vi "Rx Async.vi"(8 "error in (no error)":errorcluster, 10 "Dispatcher Interface in":refnum<class "Dispatcher Interface.lvclass">, 11 "Plugin in":refnum<class "Plugin.lvclass">) -> (0 "error out":errorcluster, 2 "Dispatcher Interface out":refnum<class "Dispatcher Interface.lvclass">, 3 "Plugin out":refnum<class "Plugin.lvclass">)   [LabVIEW 2017, in "DSF Core.lvlib" / "Plugin.lvclass"]
uses:
  Plugin.lvclass
  Interfaces/Dispatcher/Dispatcher Interface.lvclass
  C:/Git/DSF/Data Sharing Framework Core/Classes/Interfaces/Interface/Interface.lvclass
  Plugin.lvclass/Plugin.ctl
  Transfer Group/Transfer Group.lvclass/Transfer Group.ctl
  Timing/Timing.lvclass/Timing.ctl
  Interfaces/Dispatcher/Command.ctl
  Buffers/Buffers.lvclass/Buffers.ctl
  Interfaces/Interface/Interface.lvclass/Interface.ctl
  Interfaces/Dispatcher/Send Dispatcher Command.vi
  Transfer Group/Retrieve from FIFO.vi
  Transfer Group Status/Write Status.vi
  Interfaces/Dispatcher/Write.vi
  Interfaces/Dispatcher/Write Dispatcher Command.vi
  Transfer Group/Read Return FIFO.vi
  Transfer Group/Increment Late Count.vi
  Transfer Group Status/Status Size.vi
  Interfaces/Interface/Send Command.vi
  Interfaces/Interface/Write RT FIFO.vi
  Buffer/Buffer.lvclass
  C:/Git/DSF/LabVIEW-Memory/Source/Classes/Pointer/Pointer.lvclass
  Transfer Group Status/Status.lvclass
  LabVIEW-Memory/Source/Classes/Pointer/Get Address.vi
  LabVIEW-Memory/Source/Classes/Pointer/Check Size.vi
  LabVIEW-Memory/Source/Classes/Pointer/Check Null Pointer.vi
  Interfaces/Interface/Errors.vi
  Interfaces/Dispatcher/Command Timeout.vi
  VIs/VI Name.vi
  Interfaces/Dispatcher/Class Name.vi
  LabVIEW-Memory/Source/Classes/Pointer/Copy All.vi
  Transfer Group/Errors.vi
  Transfer Group/Return Timeout Error.vi
  Transfer Group/Invalid Iteration Error.vi
  Transfer Group/Transfer Group.lvclass
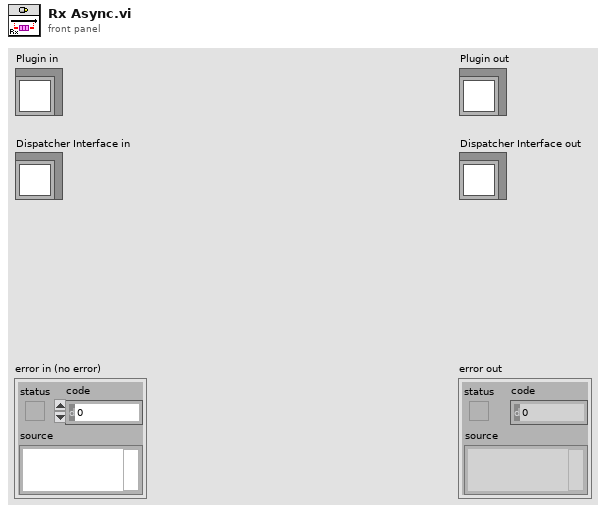
[diagram p1: front panel]
types:
  T1 = typedef "DSF Core.lvlib/Dispatcher Interface.lvclass/Command.ctl" = enum8{"Rx", "Tx", "Set Inline Buffer", "Shutdown"}
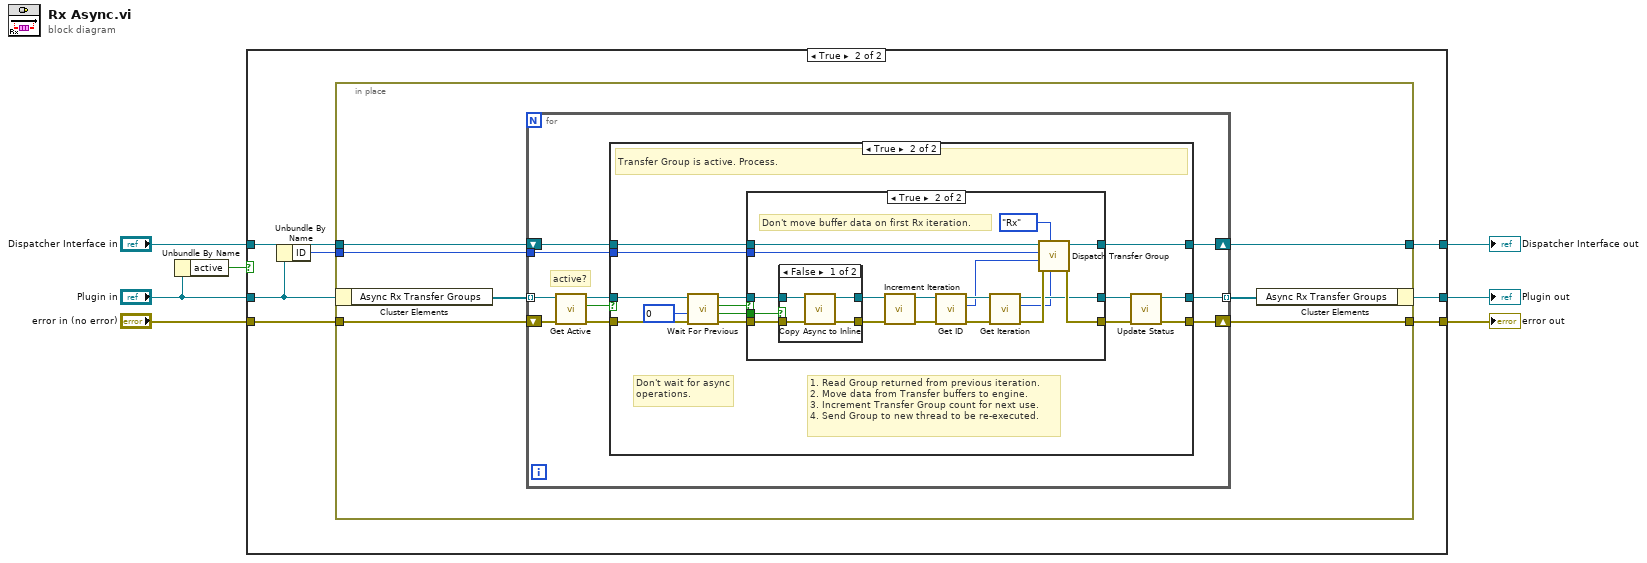
[diagram p0: block diagram]
diagram:
  n1 = Unbundle By Name("Plugin in") -> ("active"=w1:bool)
  n2 = case shown="True" w1 {
    tunnel: "error in (no error)" -> [w8 w17]
    tunnel: [w8 w16] -> w6
    tunnel: [w10 w15] -> w5
    tunnel: "Dispatcher Interface in" -> [w9 w14]
    tunnel: [w9 w13] -> w3
    tunnel: "Plugin in" -> [w10 w12]
    frame False {
    }
    frame True {
      n3 = Unbundle By Name(w12) -> ("ID"=w11:i32)
      n4 = in-place {
        in-place-border: w17 -> [w24]
        in-place-border: [w23] -> w16
        in-place-border: w14 -> [w20]
        in-place-border: [w19] -> w13
        in-place-border: w11 -> [w18]
        n5 = in-place-cluster #1(w12) -> ("Async Rx Transfer Groups"=w22:refnum<class "Transfer Group.lvclass">[])
        n6 = for {
          tunnel: w22 -> [w27] mode=indexing
          shift-right: [w33] -> w23
          shift-left: w24 -> [w32]
          tunnel: [w31] -> w21 mode=indexing
          shift-right: [w29] -> w19
          shift-left: w20 -> [w30]
          tunnel: w18 -> [w28]
          # "active?"
          n7 = call "Get Active.vi"("Transfer Group in"=w27) -> ("active"=w25:bool, "Transfer Group out"=w26:refnum<class "Transfer Group.lvclass">)  [unwired: 9 in]
          n8 = case shown="True" w25 {
            tunnel: [w36 w39] -> w33
            tunnel: w32 -> [w36 w49]
            tunnel: w26 -> [w35 w50]
            tunnel: [w35 w38] -> w31
            tunnel: w30 -> [w34 w44]
            tunnel: [w34 w45] -> w29
            tunnel: w28 -> [_ w43]
            frame False {
              # "Transfer Group is not active. Skip."
            }
            frame True {
              # "Don't wait for async operations."
              # "1. Read Group returned from previous iteration.\n2. Move data from Transfer buffers to engine.\n3. Increment Transfer Group count for next use.\n4. Send Group to new thread to be re-executed."
              # "Transfer Group is active. Process."
              n9 = call "Wait For Previous.vi"("error in (no error)"=w49, "timeout in ms (0)"=0, "Transfer Group in"=w50) -> ("error out"=w46:errorcluster, "first iteration"=w37:bool, "ready for next"=w42:bool, "Transfer Group out"=w47:refnum<class "Transfer Group.lvclass">)  [unwired: 5 in]
              n10 = case shown="True" w42 {
                tunnel: w47 -> [w53 w70]
                tunnel: [w53 w59] -> w41
                tunnel: [w52 w60] -> w40
                tunnel: w46 -> [w52 w69]
                tunnel: [w51 w57] -> w45
                tunnel: w44 -> [w51 w56]
                tunnel: w43 -> [_ w55]
                tunnel: w37 -> [_ w54]
                frame False {
                }
                frame True {
                  # "Don't move buffer data on first Rx iteration."
                  n11 = case shown="False" w54 {
                    tunnel: w70 -> [w74 w76]
                    tunnel: w69 -> [w73 w75]
                    tunnel: [w72 w76] -> w62
                    tunnel: [w71 w75] -> w61
                    frame False {
                      n12 = call "Copy Async to Inline.vi"("error in (no error)"=w73, "Transfer Group in"=w74) -> ("error out"=w71:errorcluster, "Transfer Group out"=w72:refnum<class "Transfer Group.lvclass">)  [unwired: 8 in]
                    }
                    frame True {
                    }
                  }
                  n13 = call "Increment Iteration.vi"("error in (no error)"=w61, "Transfer Group in"=w62) -> ("error out"=w66:errorcluster, "Transfer Group out"=w68:refnum<class "Transfer Group.lvclass">)  [unwired: 8 in]
                  n14 = call "Get ID.vi"("Transfer Group in"=w68) -> ("id"=w65:i32, "Transfer Group out"=w67:refnum<class "Transfer Group.lvclass">)  [unwired: 9 in]
                  n15 = call "Get Iteration.vi"("error in (no error)"=w66, "Transfer Group in"=w67) -> ("error out"=w64:errorcluster, "iteration"=w58:u64, "Transfer Group out"=w59:refnum<class "Transfer Group.lvclass">)  [unwired: 7 in]
                  n16 = call "Dispatch Transfer Group.vi"("Iteration"=w58, "command"=Command."Rx", "error in (no error)"=w64, "Transfer Group ID"=w65, "Plugin ID"=w55, "Dispatcher Interface in"=w56) -> ("error out"=w60:errorcluster, "Dispatcher Interface out"=w57:refnum<class "Dispatcher Interface.lvclass">)  [unwired: 4 in]
                }
              }
              n17 = call "Update Status.vi"("error in (no error)"=w40, "Transfer Group in"=w41) -> ("error out"=w39:errorcluster, "Transfer Group out"=w38:refnum<class "Transfer Group.lvclass">)  [unwired: 8 in]
            }
          }
        }
        n18 = in-place-cluster #1("Async Rx Transfer Groups"=w21) -> (w15:refnum<class "Plugin.lvclass">)
      }
    }
  }
  "error out" <- w6
  "Plugin out" <- w5
  "Dispatcher Interface out" <- w3
